vi "ULS Time Lapse.vi"(8 "error in (no error)":errorcluster, 9 "Time Interval(ms)":u32, 10 "Sample Count":u32, 11 "IFD in":refnum<class "IFD.lvclass">) -> (0 "error out":errorcluster, 3 "IFD out":refnum<class "IFD.lvclass">)   [LabVIEW 2016, in "IFD.lvclass"]
uses:
  IFD.lvclass
  Tag/IFD_Tag.lvclass/IFD_Tag.ctl
  IFD.lvclass/IFD.ctl
  Tag/IFD_Tag.lvclass
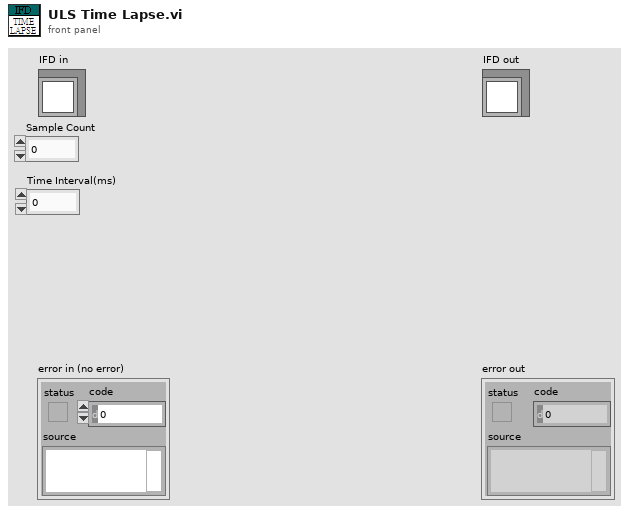
[diagram p1: front panel]
types:
  T1 = enum16{"Undefined(DO NOT USE)", "U8", "ASCII", "U16", "U32", "RATIONAL", "I8", "Undefined 8 bit", "I16", "I32", "SRATIONAL", "SGL", "DBL"}
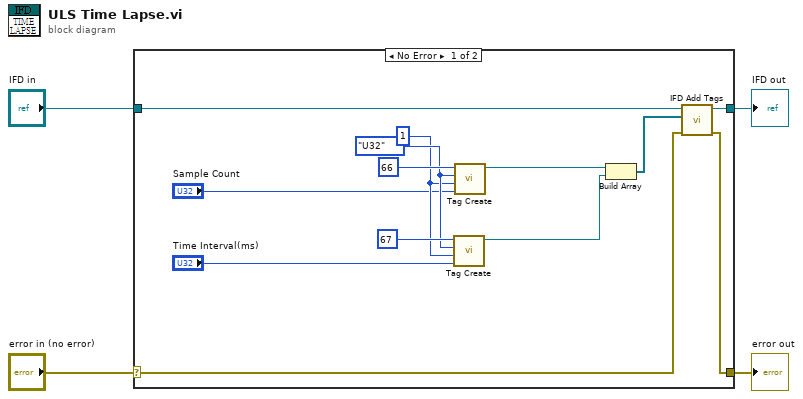
[diagram p0: block diagram]
diagram:
  n1 = case shown="No Error" "error in (no error)" {
    selector: "error in (no error)" -> [w15 w19]
    tunnel: [w14 w19] -> w3
    tunnel: [w16 w18] -> w1
    tunnel: "IFD in" -> [w17 w18]
    frame No Error {
      w7 = u32 1 ("Data Count")
      w8 = T1."U32" ("Data Type")
      n2 = call "Tag Create.vi"("Data"="Time Interval(ms)", "Data Count"=w7, "Data Type"=w8, "Tag ID"=u16 67) -> ("IFD_Tag out"=w10:refnum<class "IFD_Tag.lvclass">)  [unwired: 7 in]
      n3 = call "Tag Create.vi"("Data"="Sample Count", "Data Count"=w7, "Data Type"=w8, "Tag ID"=u16 66) -> ("IFD_Tag out"=w11:refnum<class "IFD_Tag.lvclass">)  [unwired: 7 in]
      n4 = Build Array(w11, w10) -> (w9:refnum<class "IFD_Tag.lvclass">[])
      n5 = call "IFD Add Tags.vi"("error in (no error)"=w15, "Tag(s)"=w9, "IFD in"=w17) -> ("error out"=w14:errorcluster, "IFD out"=w16:refnum<class "IFD.lvclass">)  [unwired: 7 in]
    }
    frame Error {
    }
  }
  "error out" <- w3
  "IFD out" <- w1
